vi "Component Loader Error Info.vi"(11 "error":T1) -> (3 "error info":cluster{"code":i32, "description":string})   [LabVIEW 2017, in "DSF Core.lvlib" / "Component Loader.lvclass"]
uses:
  Component Loader.lvclass
  Errors.ctl
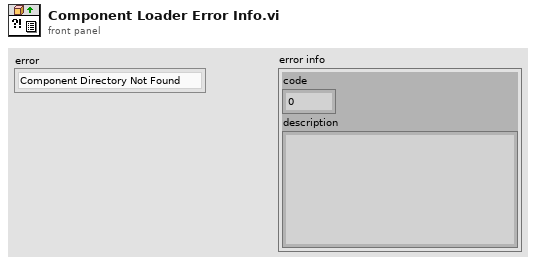
[diagram p1: front panel]
types:
  T1 = typedef "DSF Core.lvlib/Component Loader.lvclass/Errors.ctl" = enum16{"Component Directory Not Found", "Component Not Found", "Class Not Found"}
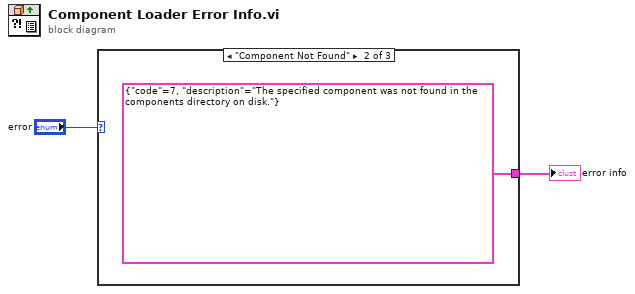
[diagram p0: block diagram]
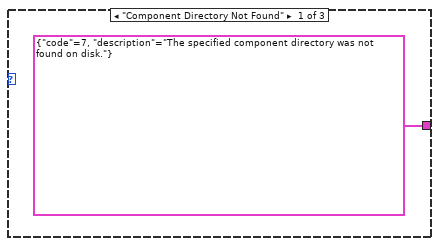
[diagram p2: hidden frame]
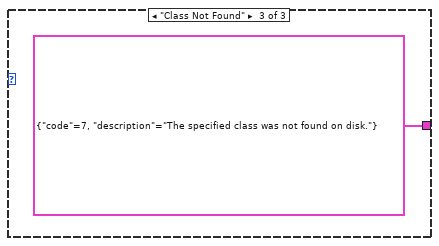
[diagram p3: hidden frame]
diagram:
  n1 = case shown="\"Component Not Found\"" "error" {
    tunnel: [cluster{"code":i32, "description":string} {"code"=7, "description"="The specified component directory was not found on disk."} cluster{"code":i32, "description":string} {"code"=7, "description"="The specified component was not found in the components directory on disk."} cluster{"code":i32, "description":string} {"code"=7, "description"="The specified class was not found on disk."}] -> w1
    frame "Component Directory Not Found" {
    }
    frame "Component Not Found" {
    }
    frame "Class Not Found" {
    }
  }
  "error info" <- w1
